vi "Local MS Auto.vi"() -> ()   [LabVIEW 2016]
uses:
  <vilib>/Platform/TimedLoop/XDataNode/timing_clust.ctl
  <vilib>/Platform/TimedLoop/XDataNode/nitl_modes.ctl
  <vilib>/Platform/TimedLoop/XDataNode/wakeup.ctl
  Subsystems/Global Variables.vi
  <vilib>/FPGAPlugInAG/PXI-7833R/niLvFpga_Open_PXI-7833R.vi
  <vilib>/Utility/error.llb/Error Cluster From Error Code.vi
  <vilib>/rvi/errors/niLvFpgaAdjustHostInterfaceError.vi
  <vilib>/Utility/file.llb/Write Delimited Spreadsheet (string).vi
  <vilib>/Utility/file.llb/Write Delimited Spreadsheet (DBL).vi
  <vilib>/FPGAPlugInAG/PXI-7833R/niLvFpga_Reset_PXI-7833R.vi
  <vilib>/FPGAPlugInAG/PXI-7833R/niLvFpga_Close_PXI-7833R.vi
  <vilib>/rvi/interface/nirviOpenFPGA/nirviOpenFPGA.xnode
  FPGA Bitfiles/PhantomControlPI_FPGATarget_QuadCtr2_E2412E44.lvbitx
  IRISS_FPGA_IO.vi
  <vilib>/rvi/interface/nirviReadWriteControl/nirviReadWriteControl.xnode
  <vilib>/platform/TimedLoop/XDataNode/XDataNode.xnode
  <vilib>/rvi/interface/nirviMethod/nirviMethod.xnode
  <vilib>/rvi/interface/nirviCloseFPGA/nirviCloseFPGA.xnode
  Library/KevinLibraryAll/labview2011/kevLib2011.lvlib
  NiFpgaLv.dll
  <vilib>/Platform/TimedLoop/XDataNode/XDNodeRunTimeDep.lvlib
panel:
  out "Pressure Reading":dbl[](array[numeric]) caption="IOP Output [mmHg]"
  in  "Pause":bool caption="To M/S"
  out "Trajectory Cluster":T1
  out "Update Mdl & Traj":bool=TRUE
  out "Stage PID Cluster":T2={"Stage Z PID"={"Kp"=0.0005, "Kd"=0.001, "Ki"=0.0}, "Stage Y PID"={"Kp"=0.0003, "Kd"=0.01, "Ki"=0.0}, "Stage X PID"={"Kp"=0.0003, "Kd"=0.01, "Ki"=0.0}}
  out "L1 to L4 PID Cluster":T3={"L1 PID Gains"={"Kp"=0.005, "Kd"=0.5, "Ki"=0.0005}, "L2 PID Gains"={"Kp"=0.01, "Kd"=1.0, "Ki"=0.0005}, "L3 PID Gains"={"Kp"=0.05, "Kd"=1.0, "Ki"=0.0005}, "L4 PID Gains"={"Kp"=0.1, "Kd"=1.0, "Ki"=0.0005}}
  in  "IRISS GUI":T4(tab)
  in  "OCT Direction":bool
  out "OCT Z out [mm]":dbl caption="OCT Out Z [mm]" format="%#.4f"
  out "X Stage out [mm] 2":dbl caption="Stage X [mm]" format="%#.4f"
  out "Z Stage out [mm] 2":dbl caption="Stage Z [mm]" format="%#.4f"
  out "Y Stage out [mm] 2":dbl caption="Stage Y [mm]" format="%#.4f"
  out "Vacuum Force [mmHg]  2":i32 caption="[mmHg]"
  out "Finished Late Counts":u16
  in  "L2 PID Gains":cluster{"Kp":dbl, "Kd":dbl, "Ki":dbl}={"Kp"=0.01, "Kd"=1.0, "Ki"=0.005}
  in  "L3 PID Gains":cluster{"Kp":dbl, "Kd":dbl, "Ki":dbl}={"Kp"=0.05, "Kd"=1.0, "Ki"=0.0005}
  in  "L4 PID Gains":cluster{"Kp":dbl, "Kd":dbl, "Ki":dbl}={"Kp"=0.1, "Kd"=0.1, "Ki"=0.0005}
  in  "L1 PID Gains":cluster{"Kp":dbl, "Kd":dbl, "Ki":dbl}={"Kp"=0.01, "Kd"=0.5, "Ki"=0.001}
  out "Current System State":T5(ring)
  out "State changing":bool
  out "Tip out Posit":dbl[](array[numeric]) caption="Position [mm]" format="%#.3f"
  out "Tip cmd Posit":dbl[](array[numeric]) caption="Command [mm]" format="%#.3f"
  out "L4 out Posit":dbl caption="y [deg]" format="%#.2g"
  out "L4 cmd Posit":dbl caption="r [deg]" format="%#.2g"
  out "L3 out Posit":dbl caption="y [mm]" format="%#.2g"
  out "L3 cmd Posit":dbl caption="r [mm]" format="%#.2g"
  out "L2 out Posit":dbl caption="y [deg]" format="%#.2g"
  out "L2 cmd Posit":dbl caption="r [deg]" format="%#.2g"
  out "L1 out Posit":dbl caption="y [deg]" format="%#.2g"
  out "L1 cmd Posit":dbl caption="r [deg]" format="%#.2g"
  out "State Flag Array":bool[](array[boolean])
  out "Irrigation Engaged? 2":bool caption="Irrigation Engaged"
  out "OCT Z cmd [mm]":dbl=6.0 caption="OCT Z Ref [mm]" min=0.0 max=12.0 step=0.5
  in  "OCT Z PID Gains":cluster{"Kp":dbl, "Kd":dbl, "Ki":dbl}={"Kp"=0.0003, "Kd"=0.0001, "Ki"=0.01}
  in  "L1 [deg]":dbl
  in  "L2 [deg]":dbl
  in  "L3 [mm]":dbl step=0.1
  in  "L4 [deg]":dbl
  in  "OCT Cmd  [mm]":dbl
  out "Current No.":u8
  in  "No. Cycles":u8=1
  in  "Joint Limits":dbl[][](array[numeric])=[[-8.0, 50.0], [-35.0, 35.0], [-5.0, 20.0], [-180.0, 180.0]] format="%#.3g"
  out "First Trk Pt":dbl[](array[numeric]) format="%#.3g"
  in  "Offset Home 2 RCM":dbl[](array[numeric])=[-7.7, 37.0, 55.0, 0.0] format="%#.3g"
  out "Error(s) Out on Program End":errorcluster
  out "L4 Chart":dbl(graph)
  out "L3 Chart":dbl(graph)
  out "L2 Chart":dbl(graph)
  out "L1 Chart":dbl(graph)
  out "Vac Input":sgl
  in  "Vacuum Step":bool
  in  "Clear Charts":bool
  out "AC Pressure [mmHg]":sgl
  out "Elaspsed Time":sgl
  in  "File Path":path=path "C:/IOPData1.txt"
  in  "Take IOP Data":bool
  out "File Exists":bool
  in  "Seconds of Data":sgl=5.0
  in  "Irrigation":bool
  in  "PID ON/OFF":bool
  in  "Vac PID Gains":cluster{"Kp":dbl, "Kd":dbl, "Ki":dbl, "Ts":dbl}={"Kp"=5.0, "Kd"=0.0, "Ki"=5.0, "Ts"=0.01}
  in  "Vac Cmd":sgl min=0 max=100 step=1 format="%#_13g"
  in  "Target IOP":sgl=20.0 min=0 max=100 step=1 format="%#_13g"
  out "IOP Ctrl":T6(graph)
  out "Pressure Sensors":T7(graph)
  in  "Reset Joystick":bool caption="Encoder Reset"
  in  "Max Limit [mmHg]":dbl=600.0
  in  "Increase":bool
  in  "Vac Step Size":sgl=50.0 min=0 max=100 step=1 format="%#_13g"
  in  "Wait Time [ms]":i32=200
  out "Vacuum":sgl
  out "Irrigation":sgl
  in  "Duty Cycle":fxp<+,32,0>
  in  "Irr Ctrl ON/OFF":bool
  in  "Hydration":bool
  in  "Pump PID Gains":cluster{"Kp":dbl, "Kd":dbl, "Ki":dbl, "Ts":dbl}={"Kp"=0.04, "Kd"=0.0, "Ki"=0.03, "Ts"=0.01}
  in  "Irr Pump Max":dbl=1.0
  in  "Height":i32
  in  "Irr Height Max":dbl=95.0
  in  "WB PID Gains":cluster{"Kp":dbl, "Kd":dbl, "Ki":dbl, "Ts":dbl}={"Kp"=0.04, "Kd"=0.0, "Ki"=0.03, "Ts"=0.01}
  out "Z Stage out [mm]":dbl caption="Output Z [mm]" format="%#.4f"
  out "Z Stage cmd [mm]":dbl=6.0 caption="Reference Z [mm]" min=0.0 max=12.0 step=0.5
  out "Y Stage out [mm]":dbl caption="Output Y [mm]" format="%#.4f"
  out "Y Stage cmd [mm]":dbl=6.0 caption="Reference Y  [mm]" min=0.0 max=12.0 step=0.5
  out "X Stage out [mm]":dbl caption="Output X [mm]" format="%#.4f"
  out "X Stage cmd [mm]":dbl=6.0 caption="Reference X [mm]" min=0.0 max=12.0 step=0.5
  in  "Stage Z PID Gains":cluster{"Kp":dbl, "Kd":dbl, "Ki":dbl}={"Kp"=0.0005, "Kd"=0.001, "Ki"=0.0}
  in  "Stage Y PID Gains":cluster{"Kp":dbl, "Kd":dbl, "Ki":dbl}={"Kp"=0.0001, "Kd"=0.005, "Ki"=0.0}
  in  "Stage X PID Gains":cluster{"Kp":dbl, "Kd":dbl, "Ki":dbl}={"Kp"=0.0003, "Kd"=0.01, "Ki"=0.0}
  out "Irrigation Engaged?":bool
  out "Accurus Button":bool[](array[boolean]) caption="Remote Button Command"
  out "Voltage Output Ch. B":dbl(graph)
  out "Voltage Output Ch. A":dbl(graph)
  out "Accurus Engaged?":bool
  out "Vacuum Force [mmHg]":i32
  in  "Load Traj":bool caption="To M/S"
  in  "Retract":bool caption="To M/S"
  in  "Stop Accurus":bool caption="To M/S"
  in  "L3 Go Home":bool caption="To M/S"
  in  "Track":bool caption="To M/S"
  in  "Program Stop":bool
  # "Robot Status"
  # "OCT"
  # "Tool Tip Location"
  # "L1"
  # "X\nY\nZ"
  # "X\nY\nZ"
  # "+"
  # "_"
  # "L2"
  # "Reserved"
  # "System Progress"
  # "L3"
  # "Homing finished"
  # "Reserved"
  # "M/S initialization finished"
  # "Trajecoty loading finished"
  # "L4"
  # "Tracking initialization finished"
  # "In Tracking"
  # "Notes: \n2. check state transition\n4. preview trajectory?"
  # "Vacuum"
  # "Joint Motion"
  # "Calibration"
  # "Space Deform Parameters"
  # "L1"
  # "[deg]"
  # "L2"
  # "[deg]"
  # "L3"
  # "[mm]"
  # "L4"
  # "[deg]"
  # "First Track Point"
  # "AC & PC Gap"
  # "L1"
  # "[deg]"
  # "L2"
  # "[deg]"
  # "L3"
  # "[mm]"
  # "L4"
  # "[deg]"
  # "Error Message"
  # "Tracking Joint Limits"
  # "Incision"
  # "Min."
  # "Max."
  # "L1"
  # "L1"
  # "[deg]"
  # "L2"
  # "L2"
  # "[deg]"
  # "L3"
  # "L3"
  # "[mm]"
  # "L4"
  # "L4"
  # "[deg]"
  # "Data Saving"
  # "Vacuum Profile"
  # "IOP Feedback Control"
  # "Eye Hydration"
  # "XYZ Stage Control"
  # "OCT Z-Axis"
  # "Moved to main tab"
  # "Foot Pedal Buttons"
  # "Irrigation and Aspiration"
  # "Button 1"
  # "Button 2"
  # "Button 3"
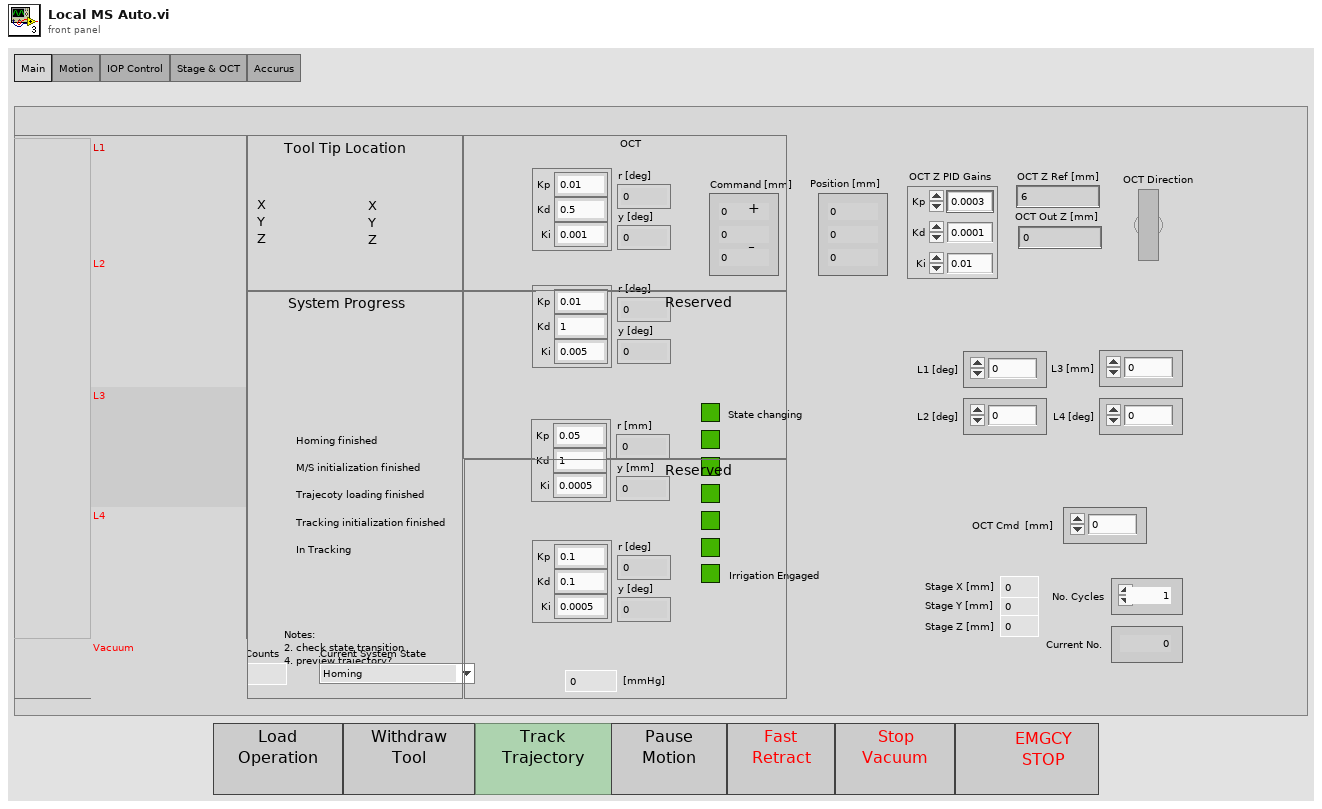
[diagram p1: front panel]
types:
  T1 = cluster{"Traj Px Array":dbl[], "Traj Py Array":dbl[], "Traj Pz Array":dbl[]}
  T2 = cluster{"Stage Z PID":cluster{"Kp":dbl, "Kd":dbl, "Ki":dbl}, "Stage Y PID":cluster{"Kp":dbl, "Kd":dbl, "Ki":dbl}, "Stage X PID":cluster{"Kp":dbl, "Kd":dbl, "Ki":dbl}}
  T3 = cluster{"L1 PID Gains":cluster{"Kp":dbl, "Kd":dbl, "Ki":dbl}, "L2 PID Gains":cluster{"Kp":dbl, "Kd":dbl, "Ki":dbl}, "L3 PID Gains":cluster{"Kp":dbl, "Kd":dbl, "Ki":dbl}, "L4 PID Gains":cluster{"Kp":dbl, "Kd":dbl, "Ki":dbl}}
  T4 = enum32{"Main", "Motion", "IOP Control", "Stage & OCT", "Accurus"}
  T5 = enum16{"Homing", "M/S Initialization", "M/S Operation", "Trajectory Loading", "Tracking Initialization", "Tracking"}
  T6 = cluster{"[0]":dbl, "[1]":dbl, "[2]":dbl, "[3]":dbl, "[4]":dbl, "[5]":dbl, "[6]":dbl, "[7]":dbl, "[8]":dbl}
  T7 = cluster{"Pressure Reading[0]":dbl, "Pressure Reading[1]":dbl, "Pressure Reading[2]":dbl, "Pressure Reading[3]":dbl, "Pressure Reading[4]":dbl, "Pressure Reading[5]":dbl, "Pressure Reading[6]":dbl, "Pressure Reading[7]":dbl, "Pressure Reading[8]":dbl}
  T8 = cluster{"Prev L1 to L4 Posit":dbl[], "Prev Stage Posit":dbl[], "Prev OCT Z Posit":dbl}
  T9 = typedef "XDNodeRunTimeDep.lvlib/timing_clust.ctl" = cluster{"Expected End [f-1]":u64, "Actual End [f-1]":u64, "Finished Late? [f-1]":bool, "Expected End [i-1]":u64, "Actual End [i-1]":u64, "Finished Late? [i-1]":bool, "Expected Start [i]":u64, "Actual Start [i]":u64, "Expected Start [f]":u64, "Actual Start [f]":u64, "Source Name":string, "Structure Name":string, "Period":i64, "Deadline":i64, "Offset":i64, "Start":i64, "Priority":i32, "Timeout":i32, "Mode":T10, "Wakeup Reason":T11, "Error":errorcluster, "Source Type":string, "Secondary Source Type":string, "Global End Time":u64, "Global Start Time":u64, "Frame Duration":u64, "Iteration Duration":u64, "Assigned CPU":i32, "I/O Scan Engine Mode":u32}
  T10 = typedef "XDNodeRunTimeDep.lvlib/nitl_modes.ctl" = enum32{"No Change", "Process missed periods, maintain original phase", "Discard missed periods, maintain original phase", "Process missed periods, ignore original phase", "Discard missed periods, ignore original phase"}
  T11 = typedef "XDNodeRunTimeDep.lvlib/wakeup.ctl" = enum32{"Normal", "Aborted", "Asynchronous wakeup", "Timing source error", "Timed loop error", "Timeout"}
  T12 = cluster{"L1 to L4 PID Cluster":cluster{"L1 PID Gains":cluster{"Kp":dbl, "Kd":dbl, "Ki":dbl}, "L2 PID Gains":cluster{"Kp":dbl, "Kd":dbl, "Ki":dbl}, "L3 PID Gains":cluster{"Kp":dbl, "Kd":dbl, "Ki":dbl}, "L4 PID Gains":cluster{"Kp":dbl, "Kd":dbl, "Ki":dbl}}, "Stage PID Cluster":cluster{"Stage Z PID":cluster{"Kp":dbl, "Kd":dbl, "Ki":dbl}, "Stage Y PID":cluster{"Kp":dbl, "Kd":dbl, "Ki":dbl}, "Stage X PID":cluster{"Kp":dbl, "Kd":dbl, "Ki":dbl}}, "OCT Z PID Gains":cluster{"Kp":dbl, "Kd":dbl, "Ki":dbl}}
  T13 = enum8{"Enabled", "Disabled", "Disabled and Grayed Out"}
  T14 = cluster{"Last L1 to L4 Posit":dbl[], "Last Stage Posit":dbl[], "Last OCT Z Posit":dbl}
  T15 = cluster{"Accurus button":bool[], "Accurus engaged?":bool, "Vacuum Force":i32, "Accurus Ch. A Vout":dbl, "Accurus Ch. B Vout":dbl, "Irrigation engaged?":bool}
  T16 = cluster{"pressure sensors[0]":sgl, "pressure sensors[1]":sgl, "pressure sensors[2]":sgl, "pressure sensors[3]":sgl, "pressure sensors[4]":sgl, "pressure sensors[5]":sgl, "pressure sensors[6]":sgl, "pressure sensors[7]":sgl, "pressure sensors[8]":sgl}[]
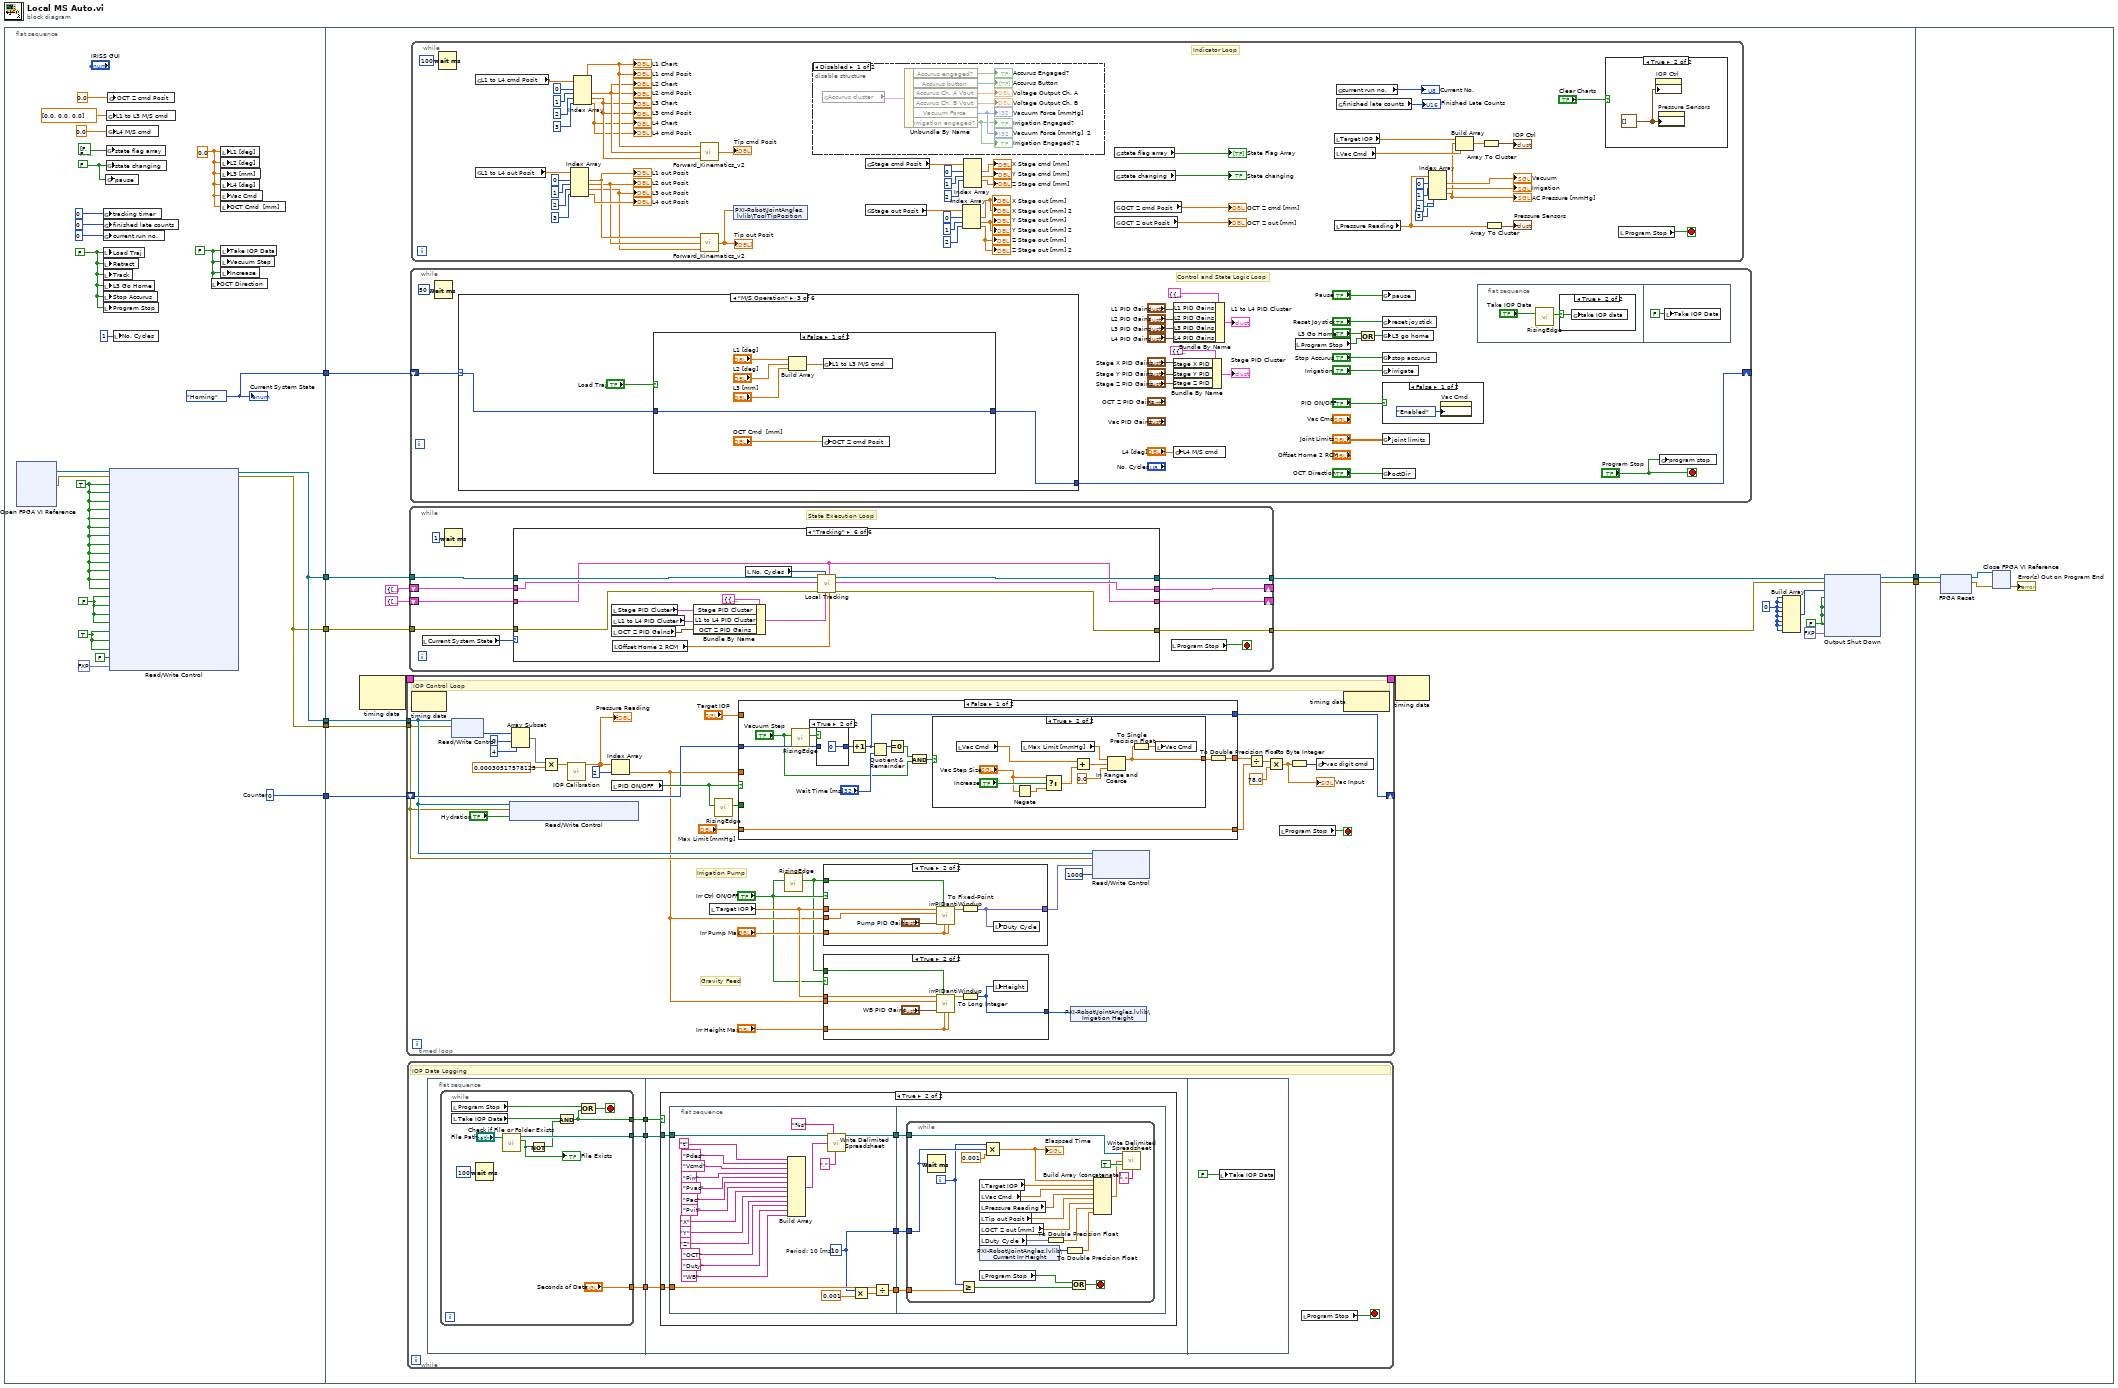
[diagram p0: block diagram]
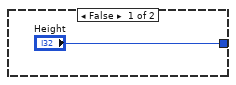
[diagram p3: hidden frame]
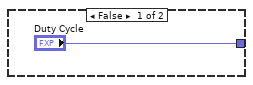
[diagram p4: hidden frame]
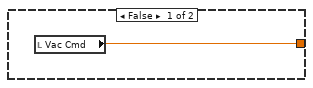
[diagram p6: hidden frame]
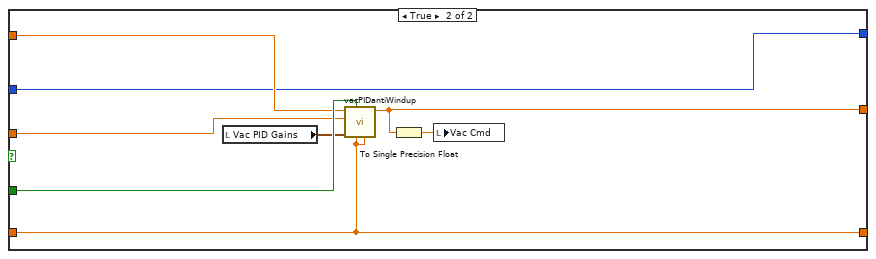
[diagram p7: hidden frame]
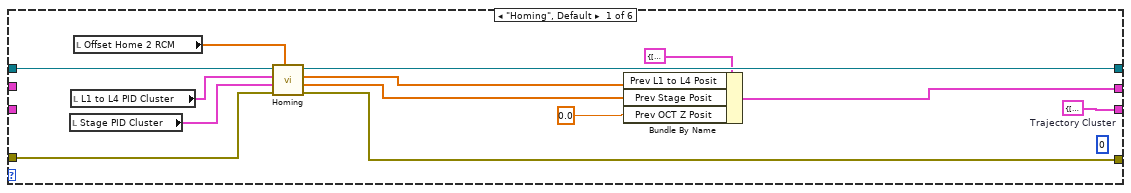
[diagram p10: hidden frame]
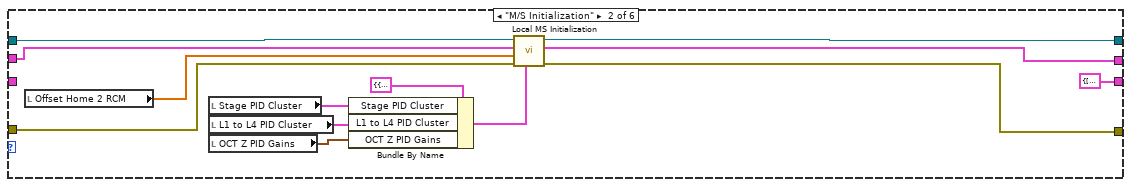
[diagram p11: hidden frame]
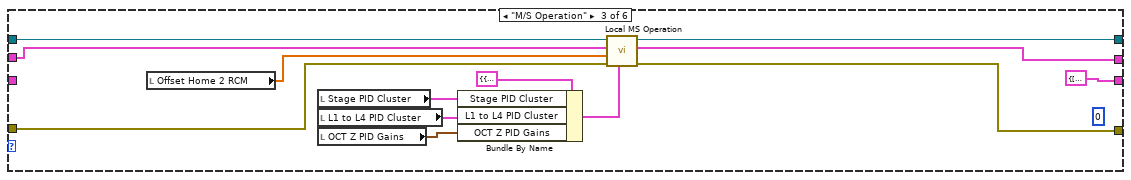
[diagram p12: hidden frame]
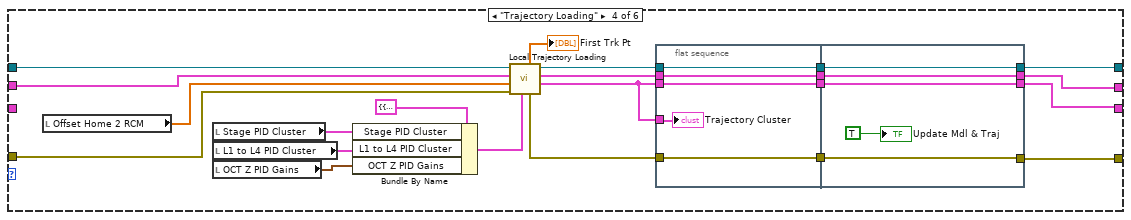
[diagram p13: hidden frame]
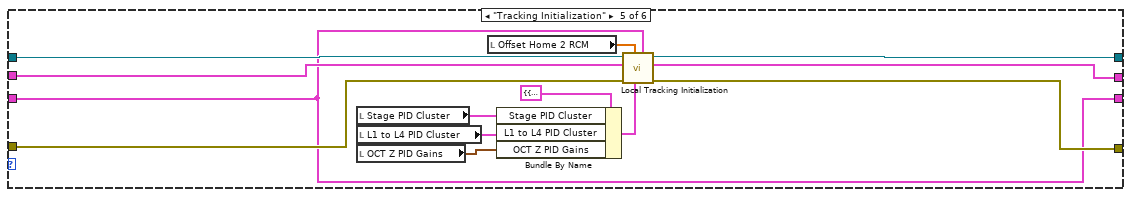
[diagram p14: hidden frame]
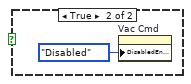
[diagram p16: hidden frame]
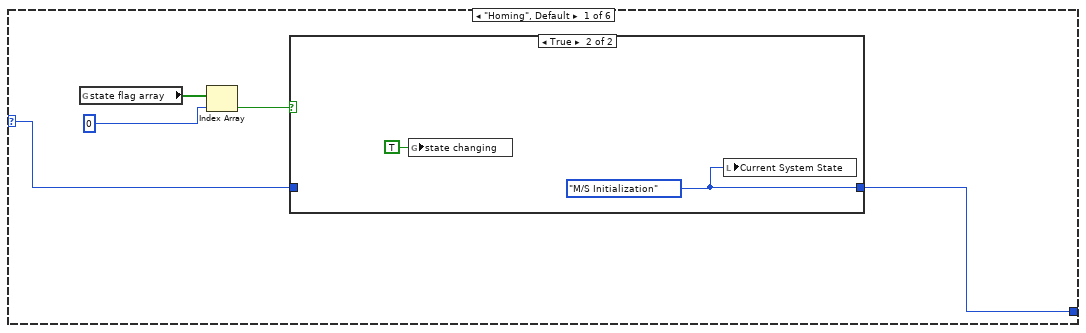
[diagram p17: hidden frame]
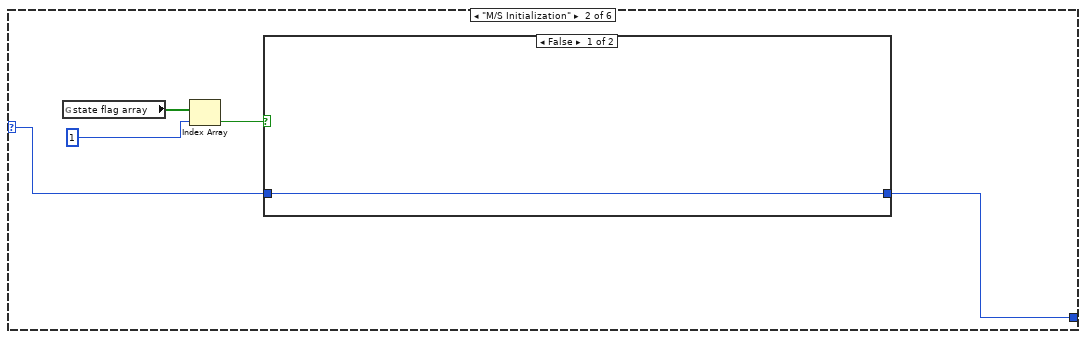
[diagram p19: hidden frame]
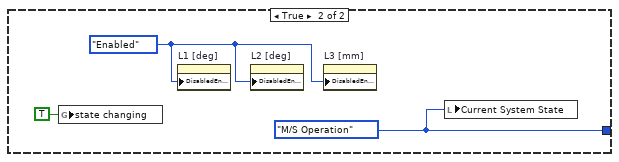
[diagram p20: hidden frame]
diagram:
  n1 = flat-sequence {
    tunnel: [w9] -> w8
    tunnel: [w10] -> w7
    tunnel: [w23] -> w6
    tunnel: [w10] -> w3
    tunnel: [w9] -> w2
    tunnel: [w15] -> w1
    tunnel: w8 -> [w48]
    tunnel: w7 -> [w49]
    tunnel: w6 -> [w40]
    tunnel: [w42] -> w5
    tunnel: [w41] -> w4
    tunnel: w3 -> [w35]
    tunnel: w2 -> [w34]
    tunnel: w1 -> [w33]
    tunnel: w5 -> [w494]
    tunnel: w4 -> [w495]
    frame #0 {
      w15 = 0  # Counter
      w12 = FALSE ("Take IOP Data")
      w13 = 0.0 ("L4 M/S cmd")
      w23 = T5."Homing" ("Current State")
      w24 = FALSE ("state changing")
      w30 = TRUE ("Conn0/DIO12 Button 1")
      w29 = FALSE ("Reset")
      w31 = TRUE ("Reset")
      w25 = FALSE ("program stop")
      n2 = xnode "Open FPGA VI Reference"() -> ("FPGA VI Reference Out"=w28:refnum<k20>, "error out"=w27:errorcluster)  [unwired: 2 in]
      n3 = global write "Global Variables.vi" "tracking timer"(0 ("finished late counts")) -> ()
      n4 = global write "Global Variables.vi" "finished late counts"(u16 0 ("finished late counts")) -> ()
      n5 = global write "Global Variables.vi" "current run no."(u8 0 ("current run no.")) -> ()
      n6 = local write "Load Traj"(w25) -> ()
      n7 = local write "Retract"(w25) -> ()
      n8 = local write "Track"(w25) -> ()
      n9 = local write "L3 Go Home"(w25) -> ()
      n10 = local write "Stop Accurus"(w25) -> ()
      n11 = local write "Program Stop"(w25) -> ()
      n12 = global write "Global Variables.vi" "pause"(w24) -> ()
      n13 = global write "Global Variables.vi" "state flag array"(bool[] [FALSE, FALSE, FALSE, FALSE, FALSE, FALSE, FALSE, FALSE, FALSE] ("state flag array")) -> ()
      n14 = global write "Global Variables.vi" "state changing"(w24) -> ()
      n15 = global write "Global Variables.vi" "L1 to L3 M/S cmd"(dbl[] [0.0, 0.0, 0.0] ("L1 to L3 M/S cmd")) -> ()
      n16 = global write "Global Variables.vi" "L4 M/S cmd"(0.0 ("L4 M/S cmd")) -> ()
      n17 = global write "Global Variables.vi" "OCT Z cmd Posit"(0.0 ("L4 M/S cmd")) -> ()
      n18 = xnode "Read/Write Control"("FPGA VI Reference In"=w28, "error in"=w27, "Reset 1"=w31, "Reset 3"=w31, "Reset 9"=w31, "Reset 10"=w31, "Reset 11"=w31, "Reset 12"=w31, "Reset 13"=w31, "Reset 14"=w31, "Reset 15"=w31, "Reset 16"=w31, "Reset 17"=w31, "Reset C1-1"=w31, "Reset C1-4"=w31, "INHB X"=w29, "INHB Y"=w29, "INHB Z"=w29, "INHB OCT Mot"=w29, "Conn0/DIO12 Button 1"=w30, "Conn0/DIO13 Button 2"=w30, "Conn0/DIO15 Button 4"=w30, "Hydration On/Off (Connector2/DIO28)"=FALSE, "Duty Cycle"=fxp<+,32,0> 0.0) -> ("FPGA VI Reference Out"=w10:refnum<k20>, "error out"=w9:errorcluster)
      n19 = local write "No. Cycles"(1 ("No. Cycles")) -> ()
      n20 = local write "OCT Direction"(w12) -> ()
      n21 = local write "L1 [deg]"(w13) -> ()
      n22 = local write "L2 [deg]"(w13) -> ()
      n23 = local write "L3 [mm]"(w13) -> ()
      n24 = local write "L4 [deg]"(w13) -> ()
      n25 = local write "Vac Cmd"(w13) -> ()
      n26 = local write "OCT Cmd  [mm]"(w13) -> ()
      n27 = local write "Take IOP Data"(w12) -> ()
      n28 = local write "Vacuum Step"(w12) -> ()
      n29 = local write "Increase"(w12) -> ()
      "Current System State" <- w23
    }
    frame #1 {
      w46 = FALSE
      w39 = i16 0 ("element")
      n30 = node-c288 ("Input Node")() -> (w37:T9)  [unwired: 2 in]
      n31 = timed-loop {
        timing: w37 -> [_]
        timing-out: [_] -> w36
        tunnel: w35 -> [w132]
        tunnel: w34 -> [w131]
        shift-right: [w135] -> _
        shift-left: w33 -> [w136]
        stop <- w146 stop-if-true
        # "Gravity Feed"
        # "Irrigation Pump"
        # "IOP Control Loop"
        n32 = node-c288() -> ()  [unwired: 1 in, 1 out]
        n33 = xnode "Read/Write Control"("FPGA VI Reference In"=w132, "error in"=w131) -> ("AI"=w149:i16[])  [unwired: 2 out]
        n34 = xnode "Read/Write Control"("FPGA VI Reference In"=w132, "error in"=w131, "Hydration On/Off (Connector2/DIO28)"="Hydration") -> ()  [unwired: 2 out]
        n35 = Array Subset(array=w149, index=0, length=4) -> (w155:i16[])
        n36 = Multiply(x=w155, y=0.00030517578125) -> (x*y=w139:dbl[])
        n37 = call "IOP Calibration.vi"("IOP Input [V]"=w139) -> ("IOP Output [mmHg]"=w150:dbl[])  [unwired: 10 in]
        "Pressure Reading" <- w150
        n38 = Index Array(array=w150, index=2) -> (element=w125:dbl)
        n39 = local read "PID ON/OFF"() -> (w147:bool)
        n40 = local read "Target IOP"() -> (w127:sgl)
        n41 = call "RisingEdge.vi"("Signal In"=w147) -> ("Rising Edge"=w148:bool)  [unwired: 10 in]
        n42 = case shown="False" w147 {
          tunnel: w125 -> [_ w200]
          tunnel: "Target IOP" -> [_ w201]
          tunnel: [w183 w204] -> w145
          tunnel: "Max Limit [mmHg]" -> [w182 w203]
          tunnel: [w182 w203] -> w137
          tunnel: w148 -> [_ w202]
          tunnel: w136 -> [w175 w197]
          tunnel: [w172 w197] -> w135
          frame False {
            n43 = call "RisingEdge.vi"("Signal In"="Vacuum Step") -> ("Rising Edge"=w176:bool)  [unwired: 10 in]
            n44 = case shown="True" w176 {
              tunnel: [w184 0] -> w179
              tunnel: w175 -> [w184 _]
              frame False {
              }
              frame True {
              }
            }
            n45 = Increment(x=w179) -> (x+1=w172:i32)
            n46 = Quotient & Remainder(x=w172, y="Wait Time [ms]") -> (x-y*floor(x/y)=w178:i32)  [unwired: 1 out]
            n47 = Equal To 0?(x=w178) -> (x = 0?=w180:bool)
            n48 = And(x=w180, y="Vacuum Step") -> (x .and. y?=w174:bool)
            n49 = case shown="True" w174 {
              tunnel: [w186 w196] -> w181
              frame False {
                n50 = local read "Vac Cmd"() -> (w186:sgl)
              }
              frame True {
                n51 = local read "Vac Cmd"() -> (w189:sgl)
                n52 = Negate(x="Vac Step Size") -> (-x=w187:sgl)
                n53 = local read "Max Limit [mmHg]"() -> (w193:dbl)
                n54 = Select(t="Vac Step Size", s="Increase", f=w187) -> (s? t:f=w191:sgl)
                n55 = Add(x=w189, y=w191) -> (x+y=w195:sgl)
                n56 = In Range and Coerce(upper limit=w193, x=w195, lower limit=0.0 ("y")) -> (coerced(x)=w196:dbl)  [unwired: 1 out]
                n57 = To Single Precision Float(number=w196) -> (single precision float=w190:sgl)
                n58 = local write "Vac Cmd"(w190) -> ()
              }
            }
            n59 = To Double Precision Float(number=w181) -> (double precision float=w183:dbl)
          }
          frame True {
            n60 = local read "Vac PID Gains"() -> (w199:cluster{"Kp":dbl, "Kd":dbl, "Ki":dbl, "Ts":dbl})
            n61 = call "vacPIDantiWindup.vi"("Saturation U"=w203, "Saturation M"=w203, "Reset"=w202, "PID Gains"=w199, "Feedback"=w200, "Reference"=w201) -> ("Control"=w204:dbl)  [unwired: 5 in]
            n62 = To Single Precision Float(number=w204) -> (single precision float=w198:sgl)
            n63 = local write "Vac Cmd"(w198) -> ()
          }
        }
        n64 = call "RisingEdge.vi"("Signal In"="Irr Ctrl ON/OFF") -> ("Rising Edge"=w123:bool)  [unwired: 10 in]
        n65 = case shown="True" "Irr Ctrl ON/OFF" {
          tunnel: ["Height" w162] -> w128
          tunnel: w127 -> [_ w159]
          tunnel: "Irr Height Max" -> [_ w161]
          tunnel: w125 -> [_ w160]
          tunnel: w123 -> [_ w158]
          frame False {
          }
          frame True {
            n66 = call "irrPIDantiWindup.vi"("Saturation U"=w161, "Saturation M"=w161, "Reset"=w158, "PID Gains"="WB PID Gains", "Feedback"=w160, "Reference"=w159) -> ("Control"=w163:dbl)  [unwired: 5 in]
            n67 = To Long Integer(number=w163) -> (32bit integer=w162:i32)
            n68 = local write "Height"(w162) -> ()
          }
        }
        n69 = case shown="True" "Irr Ctrl ON/OFF" {
          tunnel: w123 -> [_ w170]
          tunnel: w127 -> [_ w169]
          tunnel: w125 -> [_ w168]
          tunnel: ["Duty Cycle" w165] -> w130
          tunnel: "Irr Pump Max" -> [_ w166]
          frame False {
          }
          frame True {
            n70 = call "irrPIDantiWindup.vi"("Saturation U"=w166, "Saturation M"=w166, "Reset"=w170, "PID Gains"="Pump PID Gains", "Feedback"=w168, "Reference"=w169) -> ("Control"=w167:dbl)  [unwired: 5 in]
            n71 = To Fixed-Point(number=w167) -> (fixed-point=w165:fxp<+/-,32,16>)  [unwired: 1 in]
            n72 = local write "Duty Cycle"(w165) -> ()
          }
        }
        n73 = shared-variable "PXI-Robot\\JointAngles.lvlib\\Irrigation Height"(w128) -> ()  [unwired: 1 in, 1 out]
        n74 = xnode "Read/Write Control"("FPGA VI Reference In"=w132, "error in"=w131, "Duty Cycle"=w130, "Period 2 (Ticks)"=u32 1000) -> ()  [unwired: 2 out]
        n75 = Divide(x=w145, y=w137) -> (x/y=w144:dbl)
        n76 = Multiply(x=w144, y=78.0) -> (x*y=w138:dbl)
        "Vac Input" <- w138
        n77 = local read "Program Stop"() -> (w146:bool)
        n78 = To Byte Integer(number=w138) -> (8bit integer=w142:i8)
        n79 = global write "Global Variables.vi" "vac digit cmd"(w142) -> ()
        n80 = node-c288() -> ()  [unwired: 1 in, 1 out]
      }
      n81 = while {
        stop <- w50 stop-if-true
        # "IOP Data Logging"
        n82 = flat-sequence {
          tunnel: [w54] -> w53
          tunnel: [w56] -> w52
          tunnel: [w55] -> w51
          tunnel: w53 -> [w69]
          tunnel: w52 -> [w68]
          tunnel: w51 -> [w67]
          frame #0 {
            n83 = while {
              tunnel: [w65] -> w56
              tunnel: ["Seconds of Data"] -> w55
              tunnel: [w63] -> w54
              stop <- w66 stop-if-true
              n84 = local read "Program Stop"() -> (w59:bool)
              n85 = local read "Take IOP Data"() -> (w62:bool)
              n86 = Wait (ms)(milliseconds to wait=u32 100) -> ()  [unwired: 1 out]
              n87 = call <vilib>:"Check if File or Folder Exists.vi"("path"="File Path") -> ("file or folder exists?"=w58:bool, "dup path"=w65:path)  [unwired: 8 in, 1 out]
              "File Exists" <- w58
              n88 = Not(x=w58) -> (.not. x?=w64:bool)
              n89 = And(x=w62, y=w64) -> (x .and. y?=w63:bool)
              n90 = Compound Arithmetic op=OR(w59, w63) -> (w66:bool)
            }
          }
          frame #1 {
            n91 = case shown="True" w69 {
              tunnel: w68 -> [_ w74]
              tunnel: w67 -> [_ w71]
              frame False {
              }
              frame True {
                n92 = flat-sequence {
                  tunnel: w74 -> [w87]
                  tunnel: [w85] -> w73
                  tunnel: [w81] -> w72
                  tunnel: w71 -> [w95]
                  tunnel: [w93] -> w70
                  tunnel: w73 -> [w100]
                  tunnel: w72 -> [w99]
                  tunnel: w70 -> [w98]
                  frame #0 {
                    w81 = 10  # Period: 10 [ms]
                    n93 = Build Array("t" ("delimiter (\\t)"), "Pdes" ("delimiter (\\t)"), "Vcmd" ("delimiter (\\t)"), "Pirr" ("delimiter (\\t)"), "Pvac" ("delimiter (\\t)"), "Pac" ("delimiter (\\t)"), "Pvit" ("delimiter (\\t)"), "X" ("delimiter (\\t)"), "Y" ("delimiter (\\t)"), "Z" ("delimiter (\\t)"), "OCT" ("delimiter (\\t)"), "Duty" ("delimiter (\\t)"), "WB" ("delimiter (\\t)")) -> (w84:string[])
                    n94 = call-poly <vilib>:"Write Delimited Spreadsheet.vi"("file path (dialog if empty)"=w87, "format (%s)"="%s", "1D data"=w84, "delimiter (\\t)"="," ("delimiter (\\t)")) -> ("new file path (Not A Path if cancelled)"=w85:path)  [unwired: 10 in, 1 out]
                    n95 = Multiply(x=w81, y=0.001) -> (x*y=w94:dbl)
                    n96 = Divide(x=w95, y=w94) -> (x/y=w93:dbl)
                  }
                  frame #1 {
                    n97 = while {
                      tunnel: w100 -> [w115]
                      tunnel: w99 -> [w119]
                      tunnel: w98 -> [w117]
                      i -> [w118]
                      stop <- w121 stop-if-true
                      n98 = Wait (ms)(milliseconds to wait=w119) -> ()  [unwired: 1 out]
                      n99 = Greater Or Equal?(x=w118, y=w117) -> (x >= y?=w116:bool)
                      n100 = local read "Target IOP"() -> (w111:sgl)
                      n101 = local read "Vac Cmd"() -> (w110:sgl)
                      n102 = local read "Pressure Reading"() -> (w109:dbl[])
                      n103 = local read "Tip out Posit"() -> (w105:dbl[])
                      n104 = local read "OCT Z out [mm]"() -> (w106:dbl)
                      n105 = local read "Duty Cycle"() -> (w104:fxp<+,32,0>)
                      n106 = shared-variable "PXI-Robot\\JointAngles.lvlib\\Current Irr Height"() -> (w102:i32)  [unwired: 1 in, 1 out]
                      n107 = local read "Program Stop"() -> (w108:bool)
                      n108 = Compound Arithmetic op=MULTIPLY(w118, w119, 0.001 ("y")) -> (w107:dbl)
                      "Elaspsed Time" <- w107
                      n109 = To Double Precision Float(number=w104) -> (double precision float=w103:dbl)
                      n110 = To Double Precision Float(number=w102) -> (double precision float=w101:dbl)
                      n111 = Compound Arithmetic op=OR(w108, w116) -> (w121:bool)
                      n112 = Build Array (concatenate)(w107, w111, w110, w109, w105, w106, w103, w101) -> (w113:dbl[])
                      n113 = call-poly <vilib>:"Write Delimited Spreadsheet.vi"("file path (dialog if empty)"=w115, "1D data"=w113, "append to file? (new file:F)"=TRUE, "delimiter (\\t)"="," ("delimiter (\\t)")) -> ()  [unwired: 10 in, 2 out]
                    }
                  }
                }
              }
            }
          }
          frame #2 {
            n114 = local write "Take IOP Data"(FALSE) -> ()
          }
        }
        n115 = local read "Program Stop"() -> (w50:bool)
      }
      n116 = while {
        tunnel: w49 -> [w281]
        tunnel: w48 -> [w280]
        tunnel: [w279] -> w44
        tunnel: [w278] -> w43
        shift-right: [w276] -> _
        shift-left: T8 {"Prev L1 to L4 Posit"=[0.0, 0.0, 0.0, 0.0], "Prev Stage Posit"=[6.0, 6.0, 6.0], "Prev OCT Z Posit"=0.0} ("Prev Posit Cluster") -> [w277]
        shift-right: [w274] -> _
        shift-left: T1 {"Traj Px Array"=[], "Traj Py Array"=[], "Traj Pz Array"=[]} ("Trajectory Cluster") -> [w273]
        stop <- w275 stop-if-true
        # "State Execution Loop"
        n117 = local read "Current System State"() -> (w282:T5)
        n118 = Wait (ms)(milliseconds to wait=u32 1) -> ()  [unwired: 1 out]
        n119 = case shown="\"Tracking\"" w282 {
          tunnel: w281 -> [w296 w309 w322 w344 w367 w381]
          tunnel: w280 -> [w295 w308 w321 w343 w366 w380]
          tunnel: [w294 w307 w320 w326 w365 w379] -> w279
          tunnel: [w293 w306 w319 w332 w364 w378] -> w278
          tunnel: w277 -> [_ w305 w318 w342 w362 w377]
          tunnel: [w292 w304 w317 w331 w363 w376] -> w276
          tunnel: [w284 T1 {"Traj Px Array"=[], "Traj Py Array"=[], "Traj Pz Array"=[]} ("Trajectory Cluster") T1 {"Traj Px Array"=[], "Traj Py Array"=[], "Traj Pz Array"=[]} ("Trajectory Cluster") w324 w355 w370] -> w274
          tunnel: w273 -> [_ _ _ _ w355 w370]
          frame "Homing", Default {
            w284 = T1 {"Traj Px Array"=[], "Traj Py Array"=[], "Traj Pz Array"=[]}  # Trajectory Cluster
            (unwired) 0 ("Last Index")
            n120 = local read "Stage PID Cluster"() -> (w288:T2)
            n121 = local read "L1 to L4 PID Cluster"() -> (w289:T3)
            n122 = local read "Offset Home 2 RCM"() -> (w291:dbl[])
            n123 = call "Homing.vi"("Offset Home 2 RCM"=w291, "error in"=w295, "Stage PID Cluster"=w288, "L1 to L4 PID Cluster"=w289, "FPGA VI Reference In"=w296) -> ("error out"=w293:errorcluster, "Last Stage Posit"=w285:dbl[], "Last L1 to L4 Posit"=w286:dbl[], "FPGA VI Reference Out"=w294:refnum<k20>)  [unwired: 3 in]
            n124 = Bundle By Name(cluster=T8 {"Prev L1 to L4 Posit"=[-0.5409, 0.04404050915429177, -1.917656453185038, 0.02068014705882353], "Prev Stage Posit"=[6.001471972029684, 5.996134588585126, 6.000298217087839], "Prev OCT Z Posit"=-0.0} ("Prev Posit Cluster"), "Prev L1 to L4 Posit"=w286, "Prev Stage Posit"=w285, "Prev OCT Z Posit"=0.0) -> (w292:T8)
          }
          frame "M/S Initialization" {
            n125 = local read "Offset Home 2 RCM"() -> (w298:dbl[])
            n126 = local read "Stage PID Cluster"() -> (w303:T2)
            n127 = local read "L1 to L4 PID Cluster"() -> (w302:T3)
            n128 = local read "OCT Z PID Gains"() -> (w301:cluster{"Kp":dbl, "Kd":dbl, "Ki":dbl})
            n129 = Bundle By Name(cluster=T12 {"L1 to L4 PID Cluster"={"L1 PID Gains"={"Kp"=0.005, "Kd"=0.5, "Ki"=0.0005}, "L2 PID Gains"={"Kp"=0.01, "Kd"=1.0, "Ki"=0.005}, "L3 PID Gains"={"Kp"=0.05, "Kd"=1.0, "Ki"=0.0005}, "L4 PID Gains"={"Kp"=0.1, "Kd"=0.1, "Ki"=0.0005}}, "Stage PID Cluster"={"Stage Z PID"={"Kp"=0.0005, "Kd"=0.001, "Ki"=0.0}, "Stage Y PID"={"Kp"=0.0003, "Kd"=0.01, "Ki"=0.0}, "Stage X PID"={"Kp"=0.0003, "Kd"=0.01, "Ki"=0.0}}, "OCT Z PID Gains"={"Kp"=0.0003, "Kd"=0.0001, "Ki"=0.01}} ("PID Cluster"), "Stage PID Cluster"=w303, "L1 to L4 PID Cluster"=w302, "OCT Z PID Gains"=w301) -> (w299:T12)
            n130 = call "Local MS Initialization.vi"("PID Cluster"=w299, "error in"=w308, "Offset Home 2 RCM"=w298, "Prev Posit Cluster"=w305, "FPGA VI Reference In"=w309) -> ("error out"=w306:errorcluster, "Last Posit Cluster"=w304:T14, "FPGA VI Reference Out"=w307:refnum<k20>)  [unwired: 4 in]
          }
          frame "M/S Operation" {
            (unwired) 0 ("Last Index")
            n131 = local read "Offset Home 2 RCM"() -> (w311:dbl[])
            n132 = local read "Stage PID Cluster"() -> (w316:T2)
            n133 = local read "L1 to L4 PID Cluster"() -> (w315:T3)
            n134 = local read "OCT Z PID Gains"() -> (w314:cluster{"Kp":dbl, "Kd":dbl, "Ki":dbl})
            n135 = Bundle By Name(cluster=T12 {"L1 to L4 PID Cluster"={"L1 PID Gains"={"Kp"=0.005, "Kd"=0.5, "Ki"=0.0005}, "L2 PID Gains"={"Kp"=0.01, "Kd"=1.0, "Ki"=0.005}, "L3 PID Gains"={"Kp"=0.05, "Kd"=1.0, "Ki"=0.0005}, "L4 PID Gains"={"Kp"=0.1, "Kd"=0.1, "Ki"=0.0005}}, "Stage PID Cluster"={"Stage Z PID"={"Kp"=0.0005, "Kd"=0.001, "Ki"=0.0}, "Stage Y PID"={"Kp"=0.0003, "Kd"=0.01, "Ki"=0.0}, "Stage X PID"={"Kp"=0.0003, "Kd"=0.01, "Ki"=0.0}}, "OCT Z PID Gains"={"Kp"=0.0003, "Kd"=0.0001, "Ki"=0.01}} ("PID Cluster"), "Stage PID Cluster"=w316, "L1 to L4 PID Cluster"=w315, "OCT Z PID Gains"=w314) -> (w312:T12)
            n136 = call "Local MS Operation.vi"("PID Cluster"=w312, "error in"=w321, "Offset Home 2 RCM"=w311, "Prev Posit Cluster"=w318, "FPGA VI Reference In"=w322) -> ("error out"=w319:errorcluster, "Last Posit Cluster"=w317:T14, "FPGA VI Reference Out"=w320:refnum<k20>)  [unwired: 4 in]
          }
          frame "Trajectory Loading" {
            n137 = local read "Offset Home 2 RCM"() -> (w336:dbl[])
            n138 = local read "Stage PID Cluster"() -> (w341:T2)
            n139 = local read "L1 to L4 PID Cluster"() -> (w340:T3)
            n140 = local read "OCT Z PID Gains"() -> (w339:cluster{"Kp":dbl, "Kd":dbl, "Ki":dbl})
            n141 = Bundle By Name(cluster=T12 {"L1 to L4 PID Cluster"={"L1 PID Gains"={"Kp"=0.005, "Kd"=0.5, "Ki"=0.0005}, "L2 PID Gains"={"Kp"=0.01, "Kd"=1.0, "Ki"=0.005}, "L3 PID Gains"={"Kp"=0.05, "Kd"=1.0, "Ki"=0.0005}, "L4 PID Gains"={"Kp"=0.1, "Kd"=0.1, "Ki"=0.0005}}, "Stage PID Cluster"={"Stage Z PID"={"Kp"=0.0005, "Kd"=0.001, "Ki"=0.0}, "Stage Y PID"={"Kp"=0.0003, "Kd"=0.01, "Ki"=0.0}, "Stage X PID"={"Kp"=0.0003, "Kd"=0.01, "Ki"=0.0}}, "OCT Z PID Gains"={"Kp"=0.0003, "Kd"=0.0001, "Ki"=0.01}} ("PID Cluster"), "Stage PID Cluster"=w341, "L1 to L4 PID Cluster"=w340, "OCT Z PID Gains"=w339) -> (w337:T12)
            n142 = call "Local Trajectory Loading.vi"("PID Cluster"=w337, "error in"=w343, "Offset Home 2 RCM"=w336, "Prev Posit Cluster"=w342, "FPGA VI Reference In"=w344) -> ("Trajectory Cluster"=w323:T1, "Last Posit Cluster"=w330:T14, "FPGA VI Reference Out"=w328:refnum<k20>, "error out"=w334:errorcluster, "First Trk Pt"=→"First Trk Pt":dbl[])  [unwired: 2 in]
            n143 = flat-sequence {
              tunnel: w323 -> [w349]
              tunnel: w334 -> [w348]
              tunnel: [w348] -> w333
              tunnel: w330 -> [w347]
              tunnel: [w347] -> w329
              tunnel: w328 -> [w346]
              tunnel: [w346] -> w327
              tunnel: [w345] -> w325
              tunnel: w323 -> [w345]
              tunnel: [w353] -> w332
              tunnel: w333 -> [w353]
              tunnel: [w352] -> w331
              tunnel: w329 -> [w352]
              tunnel: w327 -> [w351]
              tunnel: [w351] -> w326
              tunnel: w325 -> [w350]
              tunnel: [w350] -> w324
              frame #0 {
                "Trajectory Cluster" <- w349
              }
              frame #1 {
                "Update Mdl & Traj" <- TRUE
              }
            }
          }
          frame "Tracking Initialization" {
            n144 = local read "Stage PID Cluster"() -> (w360:T2)
            n145 = local read "L1 to L4 PID Cluster"() -> (w359:T3)
            n146 = local read "OCT Z PID Gains"() -> (w357:cluster{"Kp":dbl, "Kd":dbl, "Ki":dbl})
            n147 = local read "Offset Home 2 RCM"() -> (w361:dbl[])
            n148 = Bundle By Name(cluster=T12 {"L1 to L4 PID Cluster"={"L1 PID Gains"={"Kp"=0.005, "Kd"=0.5, "Ki"=0.0005}, "L2 PID Gains"={"Kp"=0.01, "Kd"=1.0, "Ki"=0.005}, "L3 PID Gains"={"Kp"=0.05, "Kd"=1.0, "Ki"=0.0005}, "L4 PID Gains"={"Kp"=0.1, "Kd"=0.1, "Ki"=0.0005}}, "Stage PID Cluster"={"Stage Z PID"={"Kp"=0.0005, "Kd"=0.001, "Ki"=0.0}, "Stage Y PID"={"Kp"=0.0003, "Kd"=0.01, "Ki"=0.0}, "Stage X PID"={"Kp"=0.0003, "Kd"=0.01, "Ki"=0.0}}, "OCT Z PID Gains"={"Kp"=0.0003, "Kd"=0.0001, "Ki"=0.01}} ("PID Cluster"), "Stage PID Cluster"=w360, "L1 to L4 PID Cluster"=w359, "OCT Z PID Gains"=w357) -> (w356:T12)
            n149 = call "Local Tracking Initialization.vi"("Trajectory Cluster"=w355, "PID Cluster"=w356, "Offset Home 2 RCM"=w361, "error in"=w366, "Prev Posit Cluster"=w362, "FPGA VI Reference In"=w367) -> ("error out"=w364:errorcluster, "Last Posit Cluster"=w363:T14, "FPGA VI Reference Out"=w365:refnum<k20>)  [unwired: 3 in]
          }
          frame "Tracking" {
            n150 = local read "Stage PID Cluster"() -> (w375:T2)
            n151 = local read "L1 to L4 PID Cluster"() -> (w374:T3)
            n152 = local read "OCT Z PID Gains"() -> (w373:cluster{"Kp":dbl, "Kd":dbl, "Ki":dbl})
            n153 = local read "Offset Home 2 RCM"() -> (w369:dbl[])
            n154 = Bundle By Name(cluster=T12 {"L1 to L4 PID Cluster"={"L1 PID Gains"={"Kp"=0.005, "Kd"=0.5, "Ki"=0.0005}, "L2 PID Gains"={"Kp"=0.01, "Kd"=1.0, "Ki"=0.005}, "L3 PID Gains"={"Kp"=0.05, "Kd"=1.0, "Ki"=0.0005}, "L4 PID Gains"={"Kp"=0.1, "Kd"=0.1, "Ki"=0.0005}}, "Stage PID Cluster"={"Stage Z PID"={"Kp"=0.0005, "Kd"=0.001, "Ki"=0.0}, "Stage Y PID"={"Kp"=0.0003, "Kd"=0.01, "Ki"=0.0}, "Stage X PID"={"Kp"=0.0003, "Kd"=0.01, "Ki"=0.0}}, "OCT Z PID Gains"={"Kp"=0.0003, "Kd"=0.0001, "Ki"=0.01}} ("PID Cluster"), "Stage PID Cluster"=w375, "L1 to L4 PID Cluster"=w374, "OCT Z PID Gains"=w373) -> (w371:T12)
            n155 = local read "No. Cycles"() -> (w368:u8)
            n156 = call "Local Tracking.vi"("Offset Home 2 RCM"=w369, "Trajectory Cluster"=w370, "PID Cluster"=w371, "No. Cycles"=w368, "error in"=w380, "Prev Posit Cluster"=w377, "FPGA VI Reference In"=w381) -> ("error out"=w378:errorcluster, "Last Posit Cluster"=w376:T14, "FPGA VI Reference Out"=w379:refnum<k20>)  [unwired: 2 in]
          }
        }
        n157 = local read "Program Stop"() -> (w275:bool)
      }
      n158 = while {
        shift-right: [w388] -> _
        shift-left: w40 -> [w389]
        stop <- "Program Stop" stop-if-true
        # "Control and State Logic Loop"
        n159 = Wait (ms)(milliseconds to wait=u32 50) -> ()  [unwired: 1 out]
        n160 = case shown="\"M/S Operation\"" w389 {
          selector: w389 -> [w416 w422 w433 w444 w452 w481]
          tunnel: [w415 w423 w432 w445 w453 w482] -> w388
          frame "Homing", Default {
            n161 = global read "Global Variables.vi" "state flag array"() -> (w417:bool[])
            n162 = Index Array(array=w417, index=0) -> (element=w414:bool)
            n163 = case shown="True" w414 {
              tunnel: [w419 w420] -> w415
              tunnel: w416 -> [w419 _]
              frame False {
                # "homing in process"
              }
              frame True {
                w420 = T5."M/S Initialization" ("Current State")
                # "finish homing"
                n164 = global write "Global Variables.vi" "state changing"(TRUE ("state changing")) -> ()
                n165 = local write "Current System State"(w420) -> ()
              }
            }
          }
          frame "M/S Initialization" {
            n166 = global read "Global Variables.vi" "state flag array"() -> (w425:bool[])
            n167 = Index Array(array=w425, index=1) -> (element=w424:bool)
            n168 = case shown="False" w424 {
              tunnel: [w427 w429] -> w423
              tunnel: w422 -> [w427 _]
              frame False {
              }
              frame True {
                w429 = T5."M/S Operation" ("Current State")
                w428 = T13."Enabled" ("Disabled")
                n169 = global write "Global Variables.vi" "state changing"(TRUE ("state changing")) -> ()
                n170 = property on="L1 [deg]" class="DigNum (strict)"("DisabledEnum"=w428) -> ()  [unwired: 2 in, 2 out]
                n171 = property on="L2 [deg]" class="DigNum (strict)"("DisabledEnum"=w428) -> ()  [unwired: 2 in, 2 out]
                n172 = property on="L3 [mm]" class="DigNum (strict)"("DisabledEnum"=w428) -> ()  [unwired: 2 in, 2 out]
                n173 = local write "Current System State"(w429) -> ()
              }
            }
          }
          frame "M/S Operation" {
            n174 = case shown="False" "Load Traj" {
              tunnel: w433 -> [w439 _]
              tunnel: [w439 w441] -> w432
              frame False {
                n175 = Build Array("L1 [deg]", "L2 [deg]", "L3 [mm]") -> (w437:dbl[])
                n176 = global write "Global Variables.vi" "OCT Z cmd Posit"("OCT Cmd  [mm]") -> ()
                n177 = global write "Global Variables.vi" "L1 to L3 M/S cmd"(w437) -> ()
              }
              frame True {
                w441 = T5."Trajectory Loading" ("Current State")
                w440 = T13."Disabled and Grayed Out" ("Disabled")
                n178 = global write "Global Variables.vi" "state changing"(TRUE ("state changing")) -> ()
                n179 = local write "Load Traj"(FALSE ("Load Traj")) -> ()
                n180 = property on="L1 [deg]" class="DigNum (strict)"("DisabledEnum"=w440) -> ()  [unwired: 2 in, 2 out]
                n181 = property on="L2 [deg]" class="DigNum (strict)"("DisabledEnum"=w440) -> ()  [unwired: 2 in, 2 out]
                n182 = property on="L3 [mm]" class="DigNum (strict)"("DisabledEnum"=w440) -> ()  [unwired: 2 in, 2 out]
                n183 = local write "Current System State"(w441) -> ()
              }
            }
          }
          frame "Trajectory Loading" {
            n184 = global read "Global Variables.vi" "state flag array"() -> (w447:bool[])
            n185 = Index Array(array=w447, index=2) -> (element=w446:bool)
            n186 = case shown="False" w446 {
              tunnel: [w449 w450] -> w445
              tunnel: w444 -> [w449 _]
              frame False {
              }
              frame True {
                w450 = T5."Tracking Initialization" ("Current State")
                n187 = global write "Global Variables.vi" "state changing"(TRUE ("state changing")) -> ()
                n188 = local write "Current System State"(w450) -> ()
              }
            }
          }
          frame "Tracking Initialization" {
            n189 = global read "Global Variables.vi" "state flag array"() -> (w455:bool[])
            n190 = Index Array(array=w455, index=3) -> (element=w454:bool)
            n191 = case shown="True" w454 {
              tunnel: [w457 w467] -> w453
              tunnel: w452 -> [w458 w466]
              frame False {
                n192 = local read "Retract"() -> (w459:bool)
                n193 = case shown="False" w459 {
                  tunnel: w458 -> [w460 _]
                  tunnel: [w460 w463] -> w457
                  frame False {
                  }
                  frame True {
                    w463 = T5."M/S Initialization" ("Current State")
                    n194 = global write "Global Variables.vi" "state changing"(TRUE ("state changing")) -> ()
                    n195 = local write "Retract"(FALSE ("Load Traj")) -> ()
                    n196 = local write "Current System State"(w463) -> ()
                  }
                }
              }
              frame True {
                n197 = local read "Load Traj"() -> (w468:bool)
                n198 = Build Array("Track", w468, "Retract") -> (w470:bool[])
                n199 = Boolean Array To Number(Boolean array=w470) -> (number=w469:u32)
                n200 = case shown="2" w469 {
                  tunnel: [w471 w472 w475 w478] -> w467
                  tunnel: w466 -> [w471 _ _ _]
                  frame 0, Default {
                  }
                  frame 1 {
                    w472 = T5."Tracking" ("Current State")
                    n201 = global write "Global Variables.vi" "state changing"(TRUE ("state changing")) -> ()
                    n202 = local write "Track"(FALSE ("Track")) -> ()
                    n203 = local write "Current System State"(w472) -> ()
                  }
                  frame 2 {
                    w475 = T5."Trajectory Loading" ("Current State")
                    n204 = global write "Global Variables.vi" "state changing"(TRUE ("state changing")) -> ()
                    n205 = local write "Load Traj"(FALSE ("Load Traj")) -> ()
                    n206 = local write "Current System State"(w475) -> ()
                  }
                  frame 4 {
                    w478 = T5."M/S Initialization" ("Current State")
                    n207 = global write "Global Variables.vi" "state changing"(TRUE ("state changing")) -> ()
                    n208 = local write "Retract"(FALSE ("Load Traj")) -> ()
                    n209 = local write "Current System State"(w478) -> ()
                  }
                }
              }
            }
          }
          frame "Tracking" {
            n210 = global read "Global Variables.vi" "state flag array"() -> (w484:bool[])
            n211 = Index Array(array=w484, index=4) -> (element=w483:bool)
            n212 = case shown="True" w483 {
              tunnel: [w486 w489] -> w482
              tunnel: w481 -> [w486 w488]
              frame False {
              }
              frame True {
                n213 = local read "Retract"() -> (w487:bool)
                n214 = case shown="True" w487 {
                  tunnel: [w490 w491] -> w489
                  tunnel: w488 -> [w490 _]
                  frame False {
                  }
                  frame True {
                    w491 = T5."M/S Initialization" ("Current State")
                    n215 = global write "Global Variables.vi" "state changing"(TRUE ("state changing")) -> ()
                    n216 = local write "Retract"(FALSE ("Load Traj")) -> ()
                    n217 = local write "Current System State"(w491) -> ()
                  }
                }
              }
            }
          }
        }
        n218 = Bundle By Name(cluster=T3 {"L1 PID Gains"={"Kp"=0.005, "Kd"=0.5, "Ki"=0.0005}, "L2 PID Gains"={"Kp"=0.01, "Kd"=1.0, "Ki"=0.0005}, "L3 PID Gains"={"Kp"=0.05, "Kd"=1.0, "Ki"=0.0005}, "L4 PID Gains"={"Kp"=0.1, "Kd"=1.0, "Ki"=0.0005}} ("L1 to L4 PID Cluster 2"), "L1 PID Gains"="L1 PID Gains", "L2 PID Gains"="L2 PID Gains", "L3 PID Gains"="L3 PID Gains", "L4 PID Gains"="L4 PID Gains") -> (→"L1 to L4 PID Cluster":T3)
        n219 = Bundle By Name(cluster=T2 {"Stage Z PID"={"Kp"=0.0005, "Kd"=0.001, "Ki"=0.0}, "Stage Y PID"={"Kp"=0.0003, "Kd"=0.01, "Ki"=0.0}, "Stage X PID"={"Kp"=0.0003, "Kd"=0.01, "Ki"=0.0}} ("Stage PID Cluster 2"), "Stage X PID"="Stage X PID Gains", "Stage Y PID"="Stage Y PID Gains", "Stage Z PID"="Stage Z PID Gains") -> (→"Stage PID Cluster":T2)
        n220 = global write "Global Variables.vi" "L4 M/S cmd"("L4 [deg]") -> ()
        n221 = local read "Program Stop"() -> (w391:bool)
        n222 = Or(x="L3 Go Home", y=w391) -> (x .or. y?=w392:bool)
        n223 = global write "Global Variables.vi" "pause"("Pause") -> ()
        n224 = global write "Global Variables.vi" "reset joystick"("Reset Joystick") -> ()
        n225 = global write "Global Variables.vi" "L3 go home"(w392) -> ()
        n226 = global write "Global Variables.vi" "stop accurus"("Stop Accurus") -> ()
        n227 = global write "Global Variables.vi" "irrigate"("Irrigation") -> ()
        n228 = case shown="False" "PID ON/OFF" {
          frame False {
            n229 = property on="Vac Cmd" class="DigNum (strict)"("DisabledEnum"=T13."Enabled" ("Disabled")) -> ()  [unwired: 2 in, 2 out]
          }
          frame True {
            n230 = property on="Vac Cmd" class="DigNum (strict)"("DisabledEnum"=T13."Disabled" ("Disabled")) -> ()  [unwired: 2 in, 2 out]
          }
        }
        n231 = global write "Global Variables.vi" "joint limits"("Joint Limits") -> ()
        n232 = global write "Global Variables.vi" "octDir"("OCT Direction") -> ()
        n233 = flat-sequence {
          frame #0 {
            n234 = call "RisingEdge.vi"("Signal In"="Take IOP Data") -> ("Rising Edge"=w408:bool)  [unwired: 10 in]
            n235 = case shown="True" w408 {
              selector: w408 -> [_ w410]
              frame False {
              }
              frame True {
                n236 = global write "Global Variables.vi" "take IOP data"(w410) -> ()
              }
            }
          }
          frame #1 {
            n237 = local write "Take IOP Data"(FALSE ("Take IOP Data")) -> ()
          }
        }
        n238 = global write "Global Variables.vi" "program stop"("Program Stop") -> ()
      }
      n239 = while {
        stop <- w245 stop-if-true
        # "Indicator Loop"
        n240 = Wait (ms)(milliseconds to wait=u32 100) -> ()  [unwired: 1 out]
        n241 = global read "Global Variables.vi" "L1 to L4 cmd Posit"() -> (w237:dbl[])
        n242 = global read "Global Variables.vi" "L1 to L4 out Posit"() -> (w240:dbl[])
        n243 = Index Array(array=w240, index #1=0 ("index"), index #2=1 ("index"), index #3=2 ("index"), index #4=3 ("index")) -> (element #1=w243:dbl, element #2=w242:dbl, element #3=w241:dbl, element #4=→"L4 out Posit":dbl)
        "L3 out Posit" <- w241
        "L2 out Posit" <- w242
        "L1 out Posit" <- w243
        n244 = Index Array(array=w237, index #1=0 ("index"), index #2=1 ("index"), index #3=2 ("index"), index #4=3 ("index")) -> (element #1=w219:dbl, element #2=w218:dbl, element #3=w217:dbl, element #4=→"L4 cmd Posit" →"L4 Chart":dbl)
        "L1 cmd Posit" <- w219
        "L3 cmd Posit" <- w217
        "L2 cmd Posit" <- w218
        "L2 Chart" <- w218
        "L1 Chart" <- w219
        "L3 Chart" <- w217
        n245 = call "Forward_Kinematics_v2.vi"("theta 3"=w217, "theta 2"=w218, "theta 1"=w219) -> ("position"=→"Tip cmd Posit":dbl[])
        n246 = call "Forward_Kinematics_v2.vi"("theta 3"=w241, "theta 2"=w242, "theta 1"=w243) -> ("position"=w232:dbl[])
        "Tip out Posit" <- w232
        n247 = shared-variable "PXI-Robot\\JointAngles.lvlib\\ToolTipPosition"(w232) -> ()  [unwired: 1 in, 1 out]
        n248 = disable-structure shown="Disabled" {
          frame Disabled {
            n249 = global read "Global Variables.vi" "Accurus cluster"() -> (w271:T15)
            n250 = Unbundle By Name(w271) -> ("Accurus engaged?"=→"Accurus Engaged?":bool, "Accurus button"=→"Accurus Button":bool[], "Accurus Ch. A Vout"=→"Voltage Output Ch. A":dbl, "Accurus Ch. B Vout"=→"Voltage Output Ch. B":dbl, "Vacuum Force"=→"Vacuum Force [mmHg]" →"Vacuum Force [mmHg]  2":i32, "Irrigation engaged?"=→"Irrigation Engaged?" →"Irrigation Engaged? 2":bool)
          }
          frame Enabled {
          }
        }
        n251 = global read "Global Variables.vi" "Stage cmd Posit"() -> (w238:dbl[])
        n252 = global read "Global Variables.vi" "Stage out Posit"() -> (w239:dbl[])
        n253 = Index Array(array=w239, index #1=0 ("index"), index #2=1 ("index"), index #3=2 ("index")) -> (element #1=→"X Stage out [mm]" →"X Stage out [mm] 2":dbl, element #2=→"Y Stage out [mm]" →"Y Stage out [mm] 2":dbl, element #3=→"Z Stage out [mm]" →"Z Stage out [mm] 2":dbl)
        n254 = Index Array(array=w238, index #1=0 ("index"), index #2=1 ("index"), index #3=2 ("index")) -> (element #1=→"X Stage cmd [mm]":dbl, element #2=→"Y Stage cmd [mm]":dbl, element #3=→"Z Stage cmd [mm]":dbl)  [unwired: 1 in, 1 out]
        n255 = global read "Global Variables.vi" "state flag array"() -> (→"State Flag Array":bool[])
        n256 = global read "Global Variables.vi" "state changing"() -> (→"State changing":bool)
        n257 = global read "Global Variables.vi" "OCT Z cmd Posit"() -> (→"OCT Z cmd [mm]":dbl)
        n258 = global read "Global Variables.vi" "OCT Z out Posit"() -> (→"OCT Z out [mm]":dbl)
        n259 = local read "Target IOP"() -> (w223:sgl)
        n260 = local read "Vac Cmd"() -> (w224:sgl)
        n261 = local read "Pressure Reading"() -> (w215:dbl[])
        n262 = global read "Global Variables.vi" "current run no."() -> (→"Current No.":u8)
        n263 = global read "Global Variables.vi" "finished late counts"() -> (→"Finished Late Counts":u16)
        n264 = Index Array(array=w215, index #1=0 ("index"), index #2=1 ("index"), index #3=2 ("index"), index #4=3 ("index")) -> (element #1=→"Vacuum":dbl, element #2=→"Irrigation":dbl, element #3=w209:dbl)  [unwired: 1 out]
        "AC Pressure [mmHg]" <- w209
        n265 = Build Array(w223, w209, w224) -> (w222:dbl[])
        n266 = Array To Cluster(array=w222) -> (cluster=→"IOP Ctrl":T6)
        n267 = Array To Cluster(array=w215) -> (cluster=→"Pressure Sensors":T7)
        n268 = case shown="True" "Clear Charts" {
          frame False {
          }
          frame True {
            w272 = T16 [] ("History Data")
            n269 = property on="IOP Ctrl" class="WFChart (strict)"("History Data"=w272) -> ()  [unwired: 2 in, 2 out]
            n270 = property on="Pressure Sensors" class="WFChart (strict)"("History Data"=w272) -> ()  [unwired: 2 in, 2 out]
          }
        }
        n271 = local read "Program Stop"() -> (w245:bool)
      }
      n272 = node-c288(w36) -> ()  [unwired: 1 out]
      n273 = Build Array(w39, w39, w39, w39, w39, w39, w39, w39) -> (w45:i16[])
      n274 = xnode "Output Shut Down"("FPGA VI Reference In"=w44, "error in"=w43, "AO"=w45, "INHB X"=w46, "INHB Y"=w46, "INHB Z"=w46, "INHB OCT Mot"=w46, "Duty Cycle"=fxp<+,32,0> 0.0) -> ("FPGA VI Reference Out"=w41:refnum<k20>, "error out"=w42:errorcluster)
    }
    frame #2 {
      n275 = xnode "FPGA Reset"("FPGA VI Reference In"=w495, "error in"=w494) -> ("FPGA VI Reference Out"=w498:refnum<k20>, "error out"=w497:errorcluster)
      n276 = xnode "Close FPGA VI Reference"("FPGA VI Reference In"=w498, "error in"=w497) -> ("error out"=→"Error(s) Out on Program End":errorcluster)
    }
  }
